vi "Sum to 100.vi"() -> ()   [LabVIEW 2017]
panel:
  out "Numeric":i32
  out "Value of Sum":i32
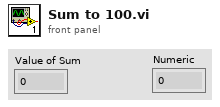
[diagram p1: front panel]
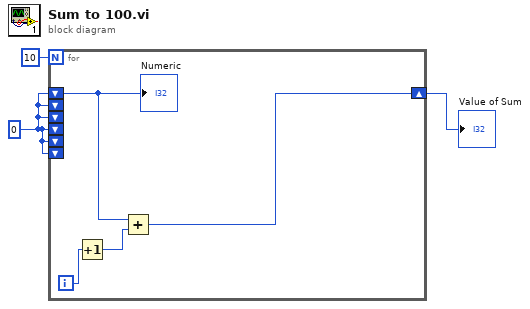
[diagram p0: block diagram]
diagram:
  w1 = 0
  n1 = for {
    N: 10 -> [_]
    shift-right: [w5] -> w2
    shift-left: w1 -> [_]
    shift-left: w1 -> [_]
    shift-left: w1 -> [_]
    shift-left: w1 -> [w4]
    shift-left: w1 -> [_]
    shift-left: w1 -> [_]
    i -> [w7]
    n2 = Increment(x=w7) -> (x+1=w6:i32)
    n3 = Add(x=w4, y=w6) -> (x+y=w5:i32)
    "Numeric" <- w4
  }
  "Value of Sum" <- w2
